vi "Distance rayon a faisceau.vi"(8 "error in (no error)":T1 caption="entrée d'erreur (pas d'erreur)", 9 "T ambiant":dbl, 10 "T max":dbl, 11 "T capteur":dbl) -> (0 "error out":T1 caption="sortie d'erreur", 3 "Rayon":dbl)   [LabVIEW 2018]
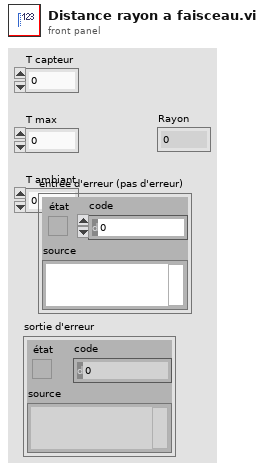
[diagram p1: front panel]
types:
  T1 = cluster{"état":bool, "code":i32, "source":string}
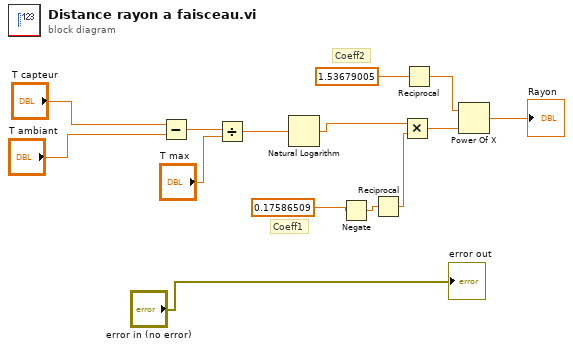
[diagram p0: block diagram]
diagram:
  # "Coeff2"
  # "Coeff1"
  n1 = Subtract(x="T capteur", y="T ambiant") -> (x-y=w12:dbl)
  n2 = Divide(x=w12, y="T max") -> (x/y=w10:dbl)
  n3 = Natural Logarithm(1:w10) -> (0:w9:dbl)
  n4 = Negate(x=0.17586509) -> (-x=w7:dbl)
  n5 = Reciprocal(x=w7) -> (1/x=w8:dbl)
  n6 = Multiply(x=w9, y=w8) -> (x*y=w4:dbl)
  n7 = Reciprocal(x=1.53679005) -> (1/x=w3:dbl)
  n8 = Power Of X(1:w4, 2:w3) -> (0:→"Rayon":dbl)
  "error out" <- "error in (no error)"
